vi "macro_Pose3d_XYZ_Axis_AngleDeg.vi"   [LabVIEW 2019, in "Trajectory_Library.lvlib"]
uses:
  Matrix_NormF.vi
  Quaternion_New.vi
  Rotation3d_Create_Default.vi
  <vilib>/Analysis/_algsub.llb/Matrix Norm.vi
  <vilib>/Analysis/_algsub.llb/Real Matrix Norm.vi
  Quaternion_New_Default.vi
  <vilib>/Analysis/Matrix/Numeric/Conversions/Array To Matrix.vi
  <vilib>/Analysis/Matrix/Numeric/Conversions/Array To Matrix - RA.vi
  Trajectory_Library.lvlib
types:
  T1 = typedef "Trajectory_Library.lvlib/ROTATION3D.ctl" = cluster{"Q_quaternion":T2}
  T2 = typedef "Trajectory_Library.lvlib/QUATERNION.ctl" = cluster{"R":dbl, "V":dbl[]}
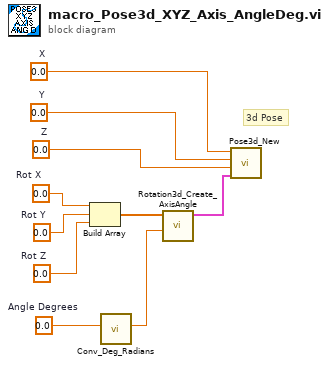
[diagram p0: block diagram]
diagram:
  w1 = 0.0  # X
  w2 = 0.0  # Y
  w3 = 0.0  # Z
  w5 = 0.0  # Angle Degrees
  w7 = 0.0  # Rot Z
  w9 = 0.0  # Rot X
  w8 = 0.0  # Rot Y
  # "3d Pose"
  n1 = Build Array(w9, w8, w7) -> (w10:dbl[])
  n2 = call "Conv_Deg_Radians.vi"("Degress"=w5) -> ("Radians"=w6:dbl)  [unwired: 10 in]
  n3 = call "Rotation3d_Create_AxisAngle.vi"("Angle"=w6, "Axis Vector"=w10) -> ("Rotation3d"=w4:T1)  [unwired: 9 in]
  n4 = call "Pose3d_New.vi"("Rotation3d"=w4, "z"=w3, "Y"=w2, "X"=w1) -> ()  [unwired: 7 in, 1 out]
